vi "WriteSLMPAttern.vi"(8 "Holo Array":T1[](array[typedef]) {"Modes"."Amplititute" step=0.05}, 11 "General settings":T2) -> (3 "Display Array":u8[][](array[numeric]))   [LabVIEW 2014]
uses:
  Controls/SLM General Settings.ctl
  Controls/Holo Settings.ctl
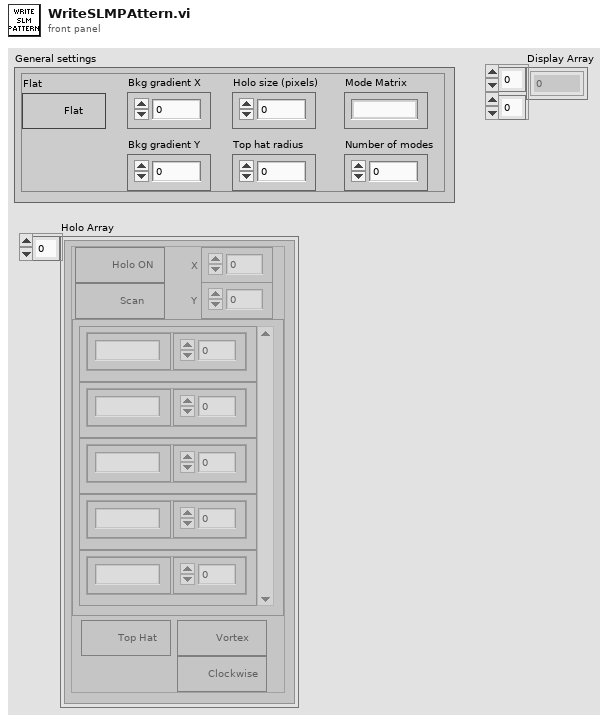
[diagram p1: front panel]
types:
  T1 = typedef "Holo Settings.ctl" = cluster{"Top Hat":bool, "Modes":cluster{"Mode ID":string, "Amplititute":dbl}[], "Vortex":bool, "Clockwise":bool, "X":dbl, "Y":dbl, "Holo ON":bool, "Scan":bool}
  T2 = typedef "SLM General Settings.ctl" = cluster{"Holo size (pixels)":i32, "Top hat radius":dbl, "Number of modes":i32, "Bkg gradient X":dbl, "Bkg gradient Y":dbl, "Flat":bool, "Mode Matrix":u16}
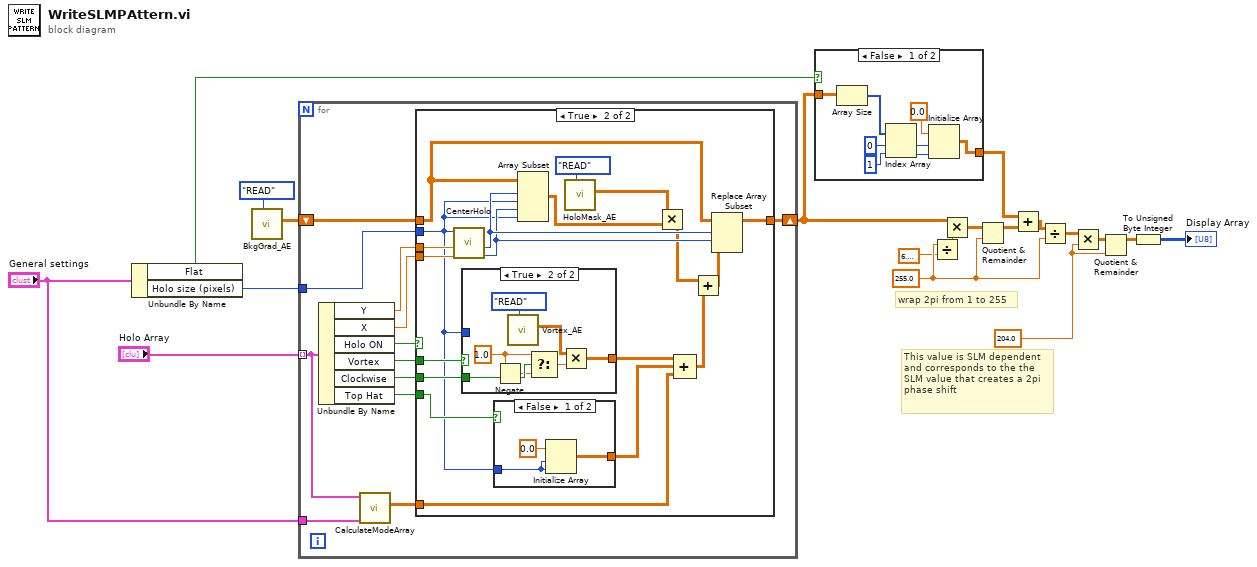
[diagram p0: block diagram]
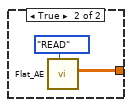
[diagram p2: hidden frame]
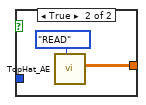
[diagram p4: hidden frame]
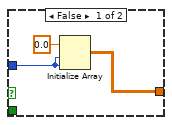
[diagram p5: hidden frame]
diagram:
  w19 = 204.0 ("Wrap Value")
  w13 = 255.0 ("y")
  # "This value is SLM dependent and corresponds to the the SLM value that creates a 2pi phase shift"
  # "wrap 2pi from 1 to 255"
  n1 = Unbundle By Name("General settings") -> ("Flat"=w9:bool, "Holo size (pixels)"=w1:i32)
  n2 = call "BkgGrad_AE.vi"("Action"=enum16{"READ", "WRITE"}."READ") -> ("BkgGrad Out"=w5:dbl[][])  [unwired: 10 in]
  n3 = for {
    tunnel: "Holo Array" -> [w21] mode=indexing
    tunnel: w1 -> [w27]
    shift-right: [w23] -> w2
    shift-left: w5 -> [w24]
    tunnel: "General settings" -> [w20]
    n4 = Unbundle By Name(w21) -> ("Y"=w26:dbl, "X"=w25:dbl, "Holo ON"=w28:bool, "Vortex"=w31:bool, "Clockwise"=w30:bool, "Top Hat"=w29:bool)
    n5 = call "CalculateModeArray.vi"("General settings"=w20, "Holo Settings"=w21) -> ("ModeArray"=w22:dbl[][])  [unwired: 9 in]
    n6 = case shown="True" w28 {
      tunnel: w31 -> [_ w47]
      tunnel: w30 -> [_ w51]
      tunnel: w24 -> [w32 w43]
      tunnel: w29 -> [_ w46]
      tunnel: w27 -> [_ w33]
      tunnel: w26 -> [_ w50]
      tunnel: w25 -> [_ w49]
      tunnel: [w32 w44] -> w23
      tunnel: w22 -> [_ w40]
      frame False {
      }
      frame True {
        n7 = call "CenterHolo.vi"("X"=w49, "Y"=w50, "Holo Size"=w33) -> ("X centered"=w41:i32, "Y centered"=w42:i32)  [unwired: 7 in]
        n8 = case shown="True" w47 {
          tunnel: w51 -> [_ w66]
          tunnel: [w58 w60] -> w39
          tunnel: w33 -> [w57 _]
          frame False {
            n9 = Initialize Array(0.0 ("element"), w57, w57) -> (w58:dbl[][])
          }
          frame True {
            w65 = 1.0 ("t")
            n10 = Negate(x=w65) -> (-x=w64:dbl)
            n11 = call "Vortex_AE.vi"("Action"=enum16{"READ", "WRITE"}."READ") -> ("Vortex Out"=w62:dbl[][])  [unwired: 10 in]
            n12 = Select(t=w65, s=w66, f=w64) -> (s? t:f=w61:dbl)
            n13 = Multiply(x=w62, y=w61) -> (x*y=w60:dbl[][])
          }
        }
        n14 = case shown="False" w46 {
          tunnel: [w53 w55] -> w45
          tunnel: w33 -> [w52 _]
          frame False {
            n15 = Initialize Array(0.0 ("element"), w52, w52) -> (w53:dbl[][])
          }
          frame True {
            n16 = call "TopHat_AE.vi"("Action"=enum16{"READ", "WRITE"}."READ") -> ("TopHat Out"=w55:dbl[][])  [unwired: 10 in]
          }
        }
        n17 = Array Subset(array=w43, index (row)=w42, length (row)=w33, index (col)=w41, length (col)=w33) -> (w34:dbl[][])
        n18 = call "HoloMask_AE.vi"("Action"=enum16{"READ", "WRITE"}."READ") -> ("HoloMask Out"=w35:dbl[][])  [unwired: 10 in]
        n19 = Multiply(x=w35, y=w34) -> (x*y=w38:dbl[][])
        n20 = Compound Arithmetic op=ADD(w39, w45, w40) -> (w36:dbl[][])
        n21 = Add(x=w38, y=w36) -> (x+y=w37:dbl[][])
        n22 = Replace Array Subset(array=w43, new element=w37, index (row)=w42, index (col)=w41) -> (w44:dbl[][])
      }
    }
  }
  n23 = case shown="False" w9 {
    tunnel: [w67 w75] -> w11
    tunnel: w2 -> [w68 _]
    frame False {
      n24 = Array Size(array=w68) -> (size(s)=w70:i32[])
      n25 = Index Array(array=w70, index #1=0 ("index"), index #2=1 ("index")) -> (element #1=w72:i32, element #2=w73:i32)
      n26 = Initialize Array(0.0 ("element"), w72, w73) -> (w67:dbl[][])
    }
    frame True {
      n27 = call "Flat_AE.vi"("Action"=enum16{"READ", "WRITE"}."READ") -> ("Flat Out"=w75:dbl[][])  [unwired: 10 in]
    }
  }
  n28 = Divide(x=w13, y=6.283185307179586) -> (x/y=w7:dbl)
  n29 = Multiply(x=w2, y=w7) -> (x*y=w6:dbl[][])
  n30 = Quotient & Remainder(x=w6, y=w13) -> (x-y*floor(x/y)=w10:dbl[][])  [unwired: 1 out]
  n31 = Add(x=w11, y=w10) -> (x+y=w12:dbl[][])
  n32 = Divide(x=w12, y=w13) -> (x/y=w14:dbl[][])
  n33 = Multiply(x=w14, y=w19) -> (x*y=w15:dbl[][])
  n34 = Quotient & Remainder(x=w15, y=w19) -> (x-y*floor(x/y)=w16:dbl[][])  [unwired: 1 out]
  n35 = To Unsigned Byte Integer(number=w16) -> (unsigned 8bit integer=→"Display Array":u8[][])
